vi "my_4th_vi.vi"() -> ()   [LabVIEW 2019]
panel:
  out "error out":errorcluster
  in  "error in (no error)":errorcluster
  out "Billard rect":T1
  in  "Color range":T2
  in  "PNG file":path
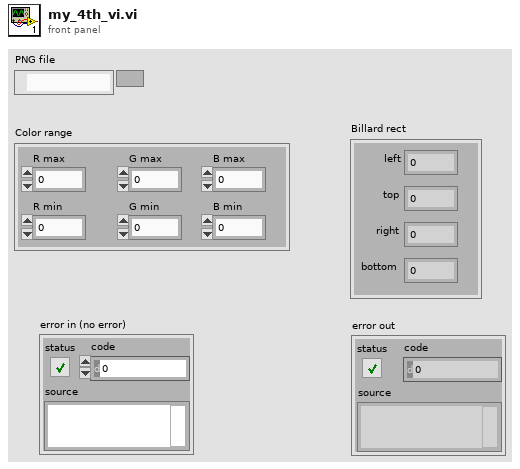
[diagram p1: front panel]
types:
  T1 = cluster{"left":i32, "top":i32, "right":i32, "bottom":i32}
  T2 = cluster{"R max":u8, "R min":u8, "G max":u8, "G min":u8, "B max":u8, "B min":u8}
  T3 = typedef "imagedata.ctl" = cluster{"image type":i32, "image depth":i32, "image":u8[], "mask":u8[], "colors":u32[], "Rectangle":cluster{"left":i16, "top":i16, "right":i16, "bottom":i16}}
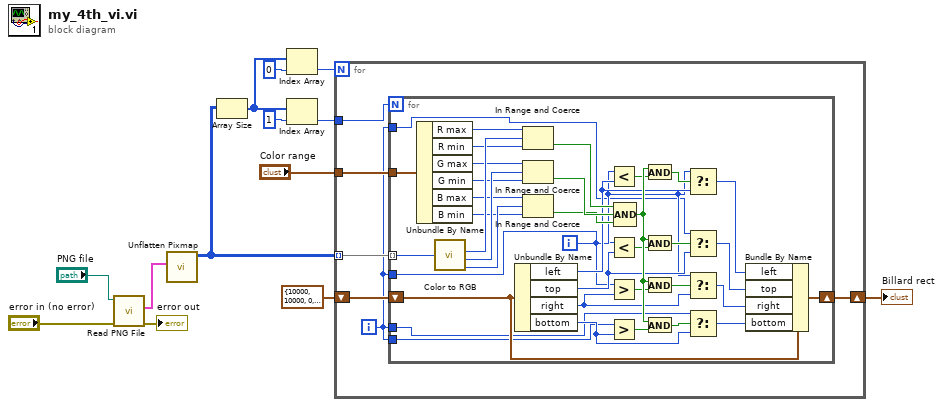
[diagram p0: block diagram]
diagram:
  n1 = call <vilib>:"Read PNG File.vi"("error in (no error)"="error in (no error)", "path to PNG file"="PNG file") -> ("error out"=→"error out":errorcluster, "image data"=w11:T3)  [unwired: 7 in, 1 out]
  n2 = call <vilib>:"Unflatten Pixmap.vi"("image data"=w11) -> ("24-bit pixmap"=w8:u32[][])  [unwired: 4 in, 6 out]
  n3 = Array Size(array=w8) -> (size(s)=w5:i32[])
  n4 = Index Array(array=w5, index=0) -> (element=w7:i32)
  n5 = Index Array(array=w5, index=1) -> (element=w3:i32)
  n6 = for {
    N: w7 -> [_]
    tunnel: w8 -> [w19] mode=indexing
    tunnel: "Color range" -> [w18]
    tunnel: w3 -> [w17]
    shift-right: [w15] -> w1
    shift-left: T1 {"left"=10000, "top"=10000, "right"=0, "bottom"=0} ("Billard rect") -> [w16]
    i -> [w14]
    n7 = for {
      N: w17 -> [_]
      tunnel: w19 -> [w57] mode=indexing
      tunnel: w18 -> [w53]
      shift-right: [w42] -> w15
      shift-left: w16 -> [w43]
      tunnel: w14 -> [w23]
      tunnel: w14 -> [w22]
      tunnel: w14 -> [w21]
      tunnel: w14 -> [w20]
      i -> [w24]
      n8 = Unbundle By Name(w53) -> ("R max"=w52:u8, "R min"=w51:u8, "G max"=w50:u8, "G min"=w49:u8, "B max"=w48:u8, "B min"=w47:u8)
      n9 = call <vilib>:"Color to RGB.vi"("Color"=w57) -> ("R"=w56:u8, "G"=w55:u8, "B"=w54:u8)  [unwired: 1 out]
      n10 = Unbundle By Name(w43) -> ("left"=w28:i32, "top"=w26:i32, "right"=w32:i32, "bottom"=w30:i32)
      n11 = In Range and Coerce(upper limit=w52, x=w56, lower limit=w51) -> (In Range?=w46:bool)  [unwired: 1 out]
      n12 = In Range and Coerce(upper limit=w50, x=w55, lower limit=w49) -> (In Range?=w45:bool)  [unwired: 1 out]
      n13 = In Range and Coerce(upper limit=w48, x=w54, lower limit=w47) -> (In Range?=w44:bool)  [unwired: 1 out]
      n14 = Less?(x=w24, y=w28) -> (x < y?=w27:bool)
      n15 = Less?(x=w20, y=w26) -> (x < y?=w25:bool)
      n16 = Greater?(x=w24, y=w32) -> (0:w31:bool)
      n17 = Greater?(x=w21, y=w30) -> (0:w29:bool)
      n18 = Compound Arithmetic op=AND(w46, w45, w44) -> (w33:bool)
      n19 = And(x=w33, y=w27) -> (x .and. y?=w41:bool)
      n20 = And(x=w33, y=w25) -> (x .and. y?=w39:bool)
      n21 = And(x=w33, y=w31) -> (x .and. y?=w37:bool)
      n22 = And(x=w33, y=w29) -> (x .and. y?=w36:bool)
      n23 = Select(t=w24, s=w41, f=w28) -> (s? t:f=w40:i32)
      n24 = Select(t=w23, s=w39, f=w26) -> (s? t:f=w38:i32)
      n25 = Select(t=w24, s=w37, f=w32) -> (s? t:f=w35:i32)
      n26 = Select(t=w22, s=w36, f=w30) -> (s? t:f=w34:i32)
      n27 = Bundle By Name(cluster=w43, "left"=w40, "top"=w38, "right"=w35, "bottom"=w34) -> (w42:T1)
    }
  }
  "Billard rect" <- w1
